vi "q2 step response.vi"() -> ()   [LabVIEW 2018]
uses:
  <vilib>/addons/Control Design/_Utility/Rendering.llb/Rendering Transfer Function Options.ctl
  <vilib>/addons/Control Design/_Model Construction/Data Typedefs.llb/CD Parametric Time Response Data.ctl
  <vilib>/addons/Control Design/_Model Construction/Data Typedefs.llb/CD MIMO Time Response Data.ctl
  <vilib>/addons/Control Design/_Model Construction/Data Typedefs.llb/CD Plot Types Enum.ctl
  <vilib>/imath/engines/lvmath/Plug In/_Char/NIMS_CH_character datatype.ctl
  <vilib>/addons/Control Design/_Model Construction/Model Creation.llb/Model Creation SubVI/cd_Create Transfer Function Model.vi
  <vilib>/addons/Control Design/_Model Conversions/Model Type.llb/Model Conversion SubVI/cd_Convert Transfer Function to State-Space Model.vi
  <vilib>/addons/Control Design/_Time Response Analysis/Time Response.llb/Time Response subVI/cd_Parametric Time Response (SS).vi
  <vilib>/addons/Control Design/_Time Response Analysis/Time Response.llb/Time Response subVI/cd_Step Response (State-Space).vi
  <vilib>/addons/Control Design/_Utility/Model Viewer.llb/Model Viewer SubVI/cd_Draw State-Space Equation (SS).vi
  <vilib>/addons/Control Design/_Utility/Model Viewer.llb/Model Viewer SubVI/cd_Draw Transfer Function Equation (TF).vi
  <vilib>/imath/engines/lvmath2/RunTimeEngine/Managers/WorkSpace/UID Generator.vi
  <vilib>/imath/engines/lvmath/Plug In/Control Design/BuiltInFunctions/tf/NIMS_CD_tf(num,den,Ts).vi
  <vilib>/imath/engines/lvmath/Plug In/Control Design/BuiltInFunctions/step/NIMS_CD_[Y,T]=step(TF,[Tinfo]).vi
  <vilib>/imath/engines/lvmath2/RunTimeEngine/BuiltInFunctions/plot/NIMS_plot(RM, RM, Str).vi
  <vilib>/imathl/engines/lvmath/Functions/Error Handling/Create Error.vi
  <vilib>/imath/engines/lvmath/Plug In/_Char/NIMS_CH_Character RV to String.vi
  <vilib>/imath/engines/lvmath2/RunTimeEngine/BuiltInFunctions/title/NIMS_title.vi
  <vilib>/imath/engines/lvmath2/RunTimeEngine/BuiltInFunctions/xlabel/NIMS_xlabel.vi
  <vilib>/imath/engines/lvmath2/RunTimeEngine/BuiltInFunctions/ylabel/NIMS_ylabel.vi
  <vilib>/imath/engines/lvmath2/RunTimeEngine/Managers/SymbolTable/Clear UID.vi
  <vilib>/imath/engines/lvmath2/RunTimeEngine/ErrorHandling/NIMS_Finalize Error.vi
  <vilib>/addons/Control Design/_Model Construction/NI_LinSys_Model Creation.lvlib
  <vilib>/addons/Control Design/_Utility/NI_CD_Model Viewer.lvlib
  <vilib>/addons/Control Design/_Model Conversions/NI_CD_Model Type.lvlib
  <vilib>/addons/Control Design/_Time Response Analysis/NI_CD_Time Response.lvlib
  <vilib>/imath/engines/lvmath2/RunTimeEngine/Managers/SymbolTable/NIMS_WorkSpace.lvlib
  <vilib>/addons/Control Design/_Utility/NI_LinSys_Rendering.lvlib
  <vilib>/addons/Control Design/_Model Construction/NI_LinSys_Data Typedefs.lvlib
panel:
  out "Time Response":cluster{"time":dbl[], dbl[]}[](graph) caption="Time Response Graph"
  out "State Trajectory Graph":cluster{"time":dbl[], dbl[]}[](graph)
  out "Step Response Data":T1={"Time"=[], "Outputs Data"=[], "States Data"=[], "plot type"=enum."step"} {"States Data" format="%#.6g"; "Outputs Data" format="%#.6g"; "Time" format="%#.6g"}
  out "Time Response Parametric Data":T3={"Rise Time (s)"=[[0.0, 0.0], [0.0, 0.0]], "Peak Time (s)"=[[16.01539885840777, 17.159355919722614], [7.372167728473419, 117.70047097528251]], "Settling Time (s)"=[[0.0, 0.0], [0.0, 0.0]], "Overshoot (%)"=[[2.6933680524159342, 1.5395749934973058], [324.8704022191171, -0.0007732741527544107]], "Steady-State Gain"=[[0.0, 0.0], [0.0, 0.0]], "Peak Value"=[[0.0, 0.0], [0.0, 0.0]]}
  out "Step Response Graph":cluster{"time":dbl[], dbl[]}[](graph)
  out "State Space":picture
  out "Transfer Function":picture
  in  "Display Format":T4 items=["Descending", "Ascending", "Negative Power"]
  in  "Denominator":dbl[](array[numeric]) format="%#.5g"
  in  "Numerator":dbl[](array[numeric]) format="%#.5g"
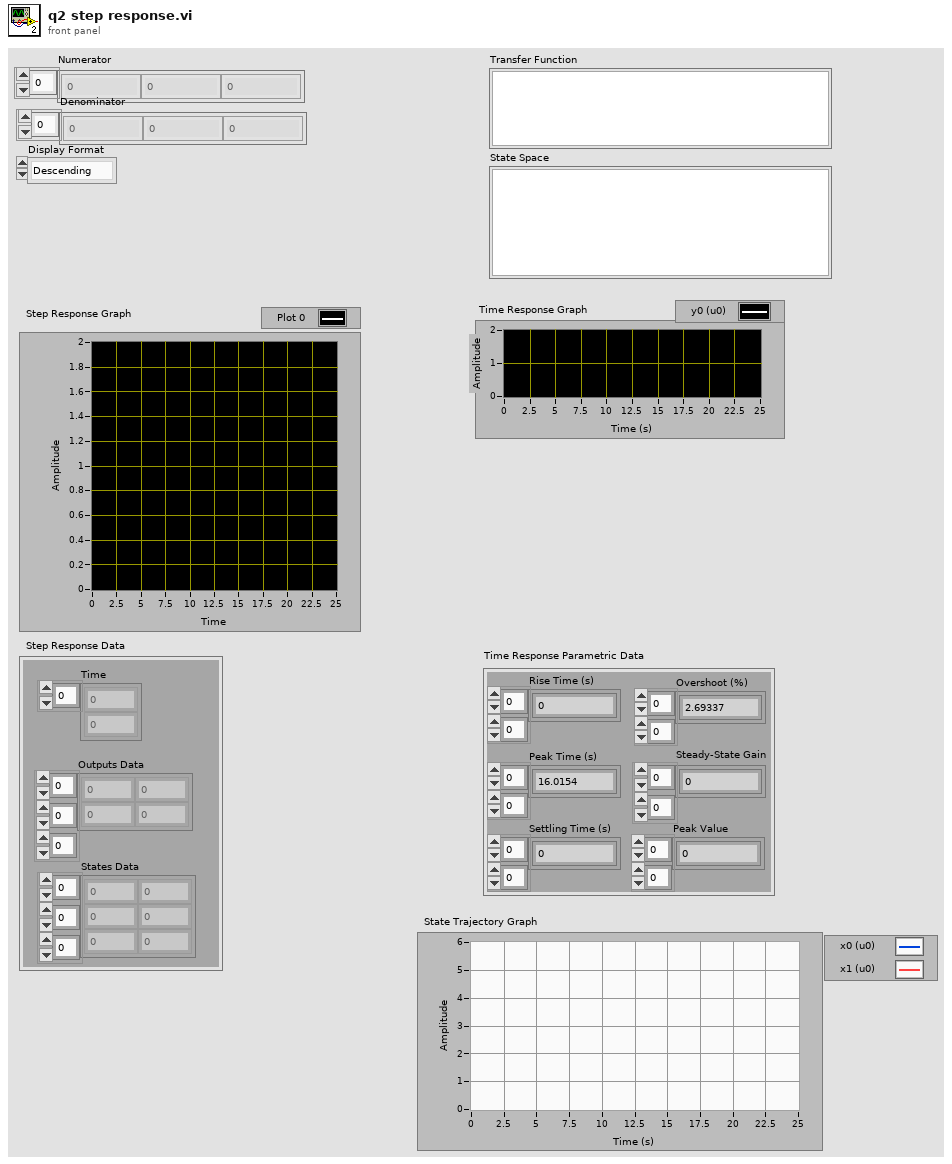
[diagram p1: front panel]
types:
  T1 = typedef "NI_LinSys_Data Typedefs.lvlib/CD MIMO Time Response Data.ctl" = cluster{"Time":dbl[], "Outputs Data":dbl[][][], "States Data":dbl[][][], "plot type":T2}
  T2 = typedef "NI_LinSys_Data Typedefs.lvlib/CD Plot Types Enum.ctl" = enum16{"bode-magnitude", "bode-phase", "nichols", "nyquist", "singular values", "step", "impulse", "initial", "simulation", "nyquist with separation"}
  T3 = typedef "NI_LinSys_Data Typedefs.lvlib/CD Parametric Time Response Data.ctl" = cluster{"Rise Time (s)":dbl[][], "Peak Time (s)":dbl[][], "Settling Time (s)":dbl[][], "Overshoot (%)":dbl[][], "Steady-State Gain":dbl[][], "Peak Value":dbl[][]}
  T4 = typedef "NI_LinSys_Rendering.lvlib/Rendering Transfer Function Options.ctl" = u16
  T5 = typedef "NI_LinSys_Model Typedefs.lvlib/CD Transfer Function Model (MIMO).ctl" = cluster{"properties":T6, "transfer function(s)":T7[][]}
  T6 = typedef "NI_LinSys_Model Typedefs.lvlib/CD General Elements.ctl" = cluster{"Model name":string, "Input names":string[], "Output names":string[], "Input Delays":dbl[], "Output Delays":dbl[], "Sampling Time":dbl, "Notes":string}
  T7 = typedef "NI_LinSys_Model Typedefs.lvlib/CD Transfer Function Model (SISO).ctl" = cluster{"Numerator":dbl[], "Denominator":dbl[], "delay":dbl}
  T8 = typedef "NI_LinSys_Model Typedefs.lvlib/CD State Space Model (MIMO).ctl" = cluster{"properties":T6, "A":dbl[][], "B":dbl[][], "C":dbl[][], "D":dbl[][], "StateNames":string[], "Transport Delay":dbl[][]}
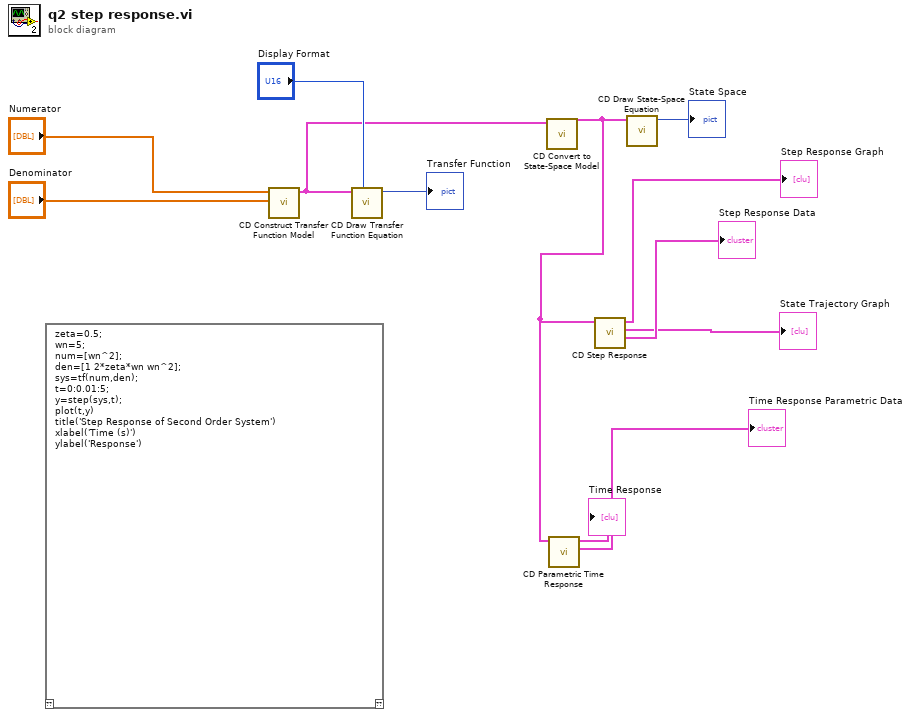
[diagram p0: block diagram]
diagram:
  n1 = mathscript code="zeta=0.5;\nwn=5;\nnum=[wn^2];\nden=[1 2*zeta*wn wn^2];\nsys=tf(num,den);\nt=0:0.01:5;\ny=step(sys,t);\nplot(t,y)\ntitle('Step Response of Second Order System')\nxlabel('Time (s)')\nylabel('Response')"() -> ()  [unwired: 1 in, 1 out]
  n2 = call-poly <vilib>:"CD Construct Transfer Function Model.vi"("Denominator"="Denominator", "Numerator"="Numerator") -> ("Transfer Function Model"=w8:T5)  [unwired: 8 in, 1 out]
  n3 = call-poly <vilib>:"CD Draw Transfer Function Equation.vi"("Display Format"="Display Format", "Transfer Function Model"=w8) -> ("Equation"=→"Transfer Function":picture)  [unwired: 7 in, 2 out]
  n4 = call-poly <vilib>:"CD Convert to State-Space Model.vi"("Transfer Function Model"=w8) -> ("State-Space Model"=w5:T8)  [unwired: 9 in, 1 out]
  n5 = call-poly <vilib>:"CD Parametric Time Response.vi"("State-Space Model"=w5) -> ("Time Response Parametric Data"=→"Time Response Parametric Data":T3, "Time Response"=→"Time Response":cluster{"time":dbl[], dbl[]}[])  [unwired: 7 in, 2 out]
  n6 = call-poly <vilib>:"CD Step Response.vi"("State-Space Model"=w5) -> ("Step Response Data"=→"Step Response Data":T1, "State Trajectory Graph"=→"State Trajectory Graph":cluster{"time":dbl[], dbl[]}[], "Step Response Graph"=→"Step Response Graph":cluster{"time":dbl[], dbl[]}[])  [unwired: 7 in, 1 out]
  n7 = call-poly <vilib>:"CD Draw State-Space Equation.vi"("State-Space Model"=w5) -> ("Equation"=→"State Space":picture)  [unwired: 8 in, 2 out]
